vi "Plot Variable.vi"() -> ()   [LabVIEW 2010]
panel:
  in  "Plot Array":dbl[](array[numeric])
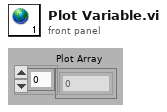
[diagram p1: front panel]
diagram:
